vi "Init Hardware.vi"(8 "error in (no error)":errorcluster, 11 "NI-Scope Lock-in Driver in":refnum<class "NI-Scope Lock-in Driver.lvclass">) -> (0 "error out":errorcluster, 3 "NI-Scope Lock-in Driver out":refnum<class "NI-Scope Lock-in Driver.lvclass">)   [LabVIEW 2016, in "NI-Scope Lock-in Driver.lvclass"]
uses:
  NI-Scope Lock-in Driver.lvclass
  C:/github/NHMFL_Core/Libraries/NI-DAQ/NI-Scope Digitizer/Ni-Scope Digitizer.lvclass
  NI-Scope Digitizer/Ni-Scope Digitizer.lvclass/Ni-Scope Digitizer.ctl
  NI-Scope Lock-in Driver.lvclass/NI-Scope Lock-in Driver.ctl
  NI-Scope Digitizer/Write Fetch Relative To.vi
  Write Sine.vi
  Write Cosine.vi
  NI-Scope Digitizer/Read instrument handle.vi
  NI-Scope Digitizer/Write instrument handle.vi
  NI-Scope Digitizer/Ni-Scope Digitizer.lvclass
  <vilib>/Analysis/NI_AALBase.lvlib
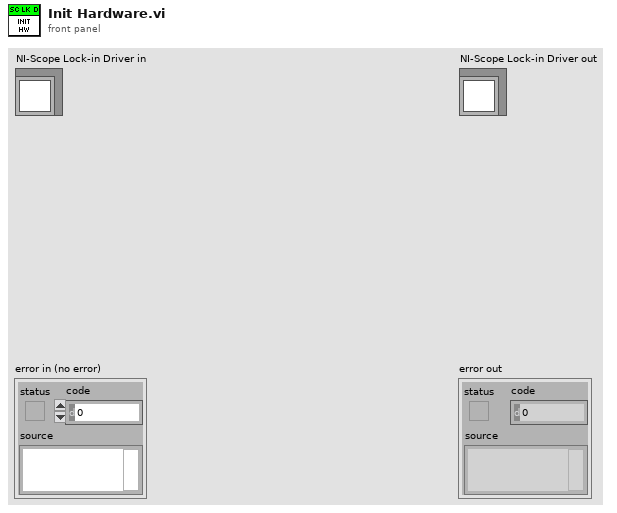
[diagram p1: front panel]
types:
  T1 = typedef "NI-Scope Lock-in Configuration.ctl" = cluster{"Pulse Configuration":T2, "Points per sine wave":i32}
  T2 = typedef "Pusle Driver Configuration.ctl" = cluster{"Pre-trigger duration":dbl, "Post-trigger duration":dbl, "Rate":dbl, "Ranges":dbl[], "Re-name channels":string[], "Active channels":string, "External clock":bool}
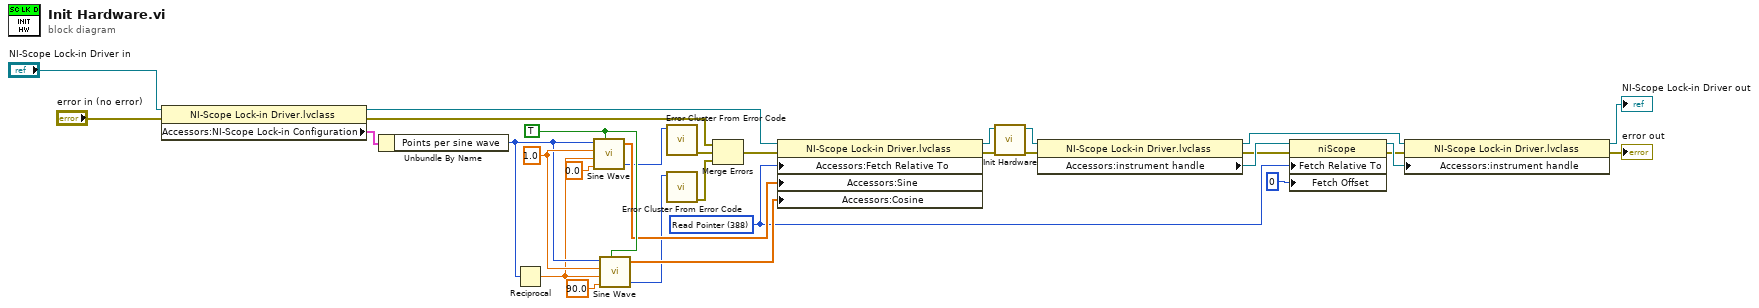
[diagram p0: block diagram]
diagram:
  w22 = 1.0
  w24 = TRUE ("reset phase")
  w8 = 388 items=["Start"=482, "Trigger"=483, "Pretrigger"=477, "Now"=481, "Read Pointer"=388] ("Fetch:Fetch Relative To")
  n1 = property class="NI-Scope Lock-in Driver.lvclass"(reference="NI-Scope Lock-in Driver in", error in="error in (no error)") -> (reference out=w26:refnum<class "NI-Scope Lock-in Driver.lvclass">, error out=w28:errorcluster, "Accessors:NI-Scope Lock-in Configuration"=w25:T1)
  n2 = Unbundle By Name(w25) -> ("Points per sine wave"=w21:i32)
  n3 = Reciprocal(x=w21) -> (1/x=w20:dbl)
  n4 = call <vilib>:"Sine Wave.vi"("samples"=w21, "amplitude"=w22, "frequency"=w20, "phase in"=0.0, "reset phase"=w24) -> ("sine wave"=w18:dbl[], "error"=w16:i32)  [unwired: 1 out]
  n5 = call <vilib>:"Sine Wave.vi"("samples"=w21, "amplitude"=w22, "frequency"=w20, "phase in"=90.0 ("y"), "reset phase"=w24) -> ("sine wave"=w17:dbl[], "error"=w15:i32)  [unwired: 1 out]
  n6 = call <vilib>:"Error Cluster From Error Code.vi"("error code (0)"=w16) -> ("error out"=w13:errorcluster)  [unwired: 8 in]
  n7 = call <vilib>:"Error Cluster From Error Code.vi"("error code (0)"=w15) -> ("error out"=w12:errorcluster)  [unwired: 8 in]
  n8 = Merge Errors(w28, w13, w12) -> (w14:errorcluster)
  n9 = property class="NI-Scope Lock-in Driver.lvclass"(reference=w26, error in=w14, "Accessors:Fetch Relative To"=w8, "Accessors:Sine"=w18, "Accessors:Cosine"=w17) -> (reference out=w29:refnum<class "NI-Scope Lock-in Driver.lvclass">, error out=w30:errorcluster)
  n10 = call-parent "Init Hardware.vi"("error in (no error)"=w30, "Ni-Scope Digitizer in"=w29) -> ("error out"=w10:errorcluster, "Ni-Scope Digitizer out"=w11:refnum<class "NI-Scope Lock-in Driver.lvclass">)  [unwired: 8 in]
  n11 = property class="NI-Scope Lock-in Driver.lvclass"(reference=w11, error in=w10) -> (reference out=w3:refnum<class "NI-Scope Lock-in Driver.lvclass">, error out=w6:errorcluster, "Accessors:instrument handle"=w9:refnum<k15>)
  n12 = property class="niScope"(reference=w9, error in=w6, "Fetch Relative To"=w8, "Fetch Offset"=0 ("Fetch:Fetch Offset")) -> (reference out=w5:refnum<k15>, error out=w4:errorcluster)
  n13 = property class="NI-Scope Lock-in Driver.lvclass"(reference=w3, error in=w4, "Accessors:instrument handle"=w5) -> (reference out=→"NI-Scope Lock-in Driver out":refnum<class "NI-Scope Lock-in Driver.lvclass">, error out=→"error out":errorcluster)
